vi "FPGA to RT to Host data stream trial.vi"() -> ()   [LabVIEW 2018]
uses:
  <vilib>/rvi/interface/nirviOpenFPGA/nirviOpenFPGA.xnode
  <vilib>/rvi/interface/nirviCloseFPGA/nirviCloseFPGA.xnode
  <vilib>/rvi/interface/nirviMethod/nirviMethod.xnode
  <vilib>/rvi/errors/niLvFpgaMergeErrorWithErrorCode.vi
  <vilib>/rvi/interface/nirviReadWriteControl/nirviReadWriteControl.xnode
  <vilib>/Utility/error.llb/Error Cluster From Error Code.vi
  <vilib>/rvi/interface/Simulation/niFpgaSimulationCallBeginRW.vi
  <vilib>/rvi/errors/niLvFpgaAdjustHostInterfaceError.vi
  <resource>/objmgr/ni.dex.rc
  <vilib>/dex/Flush And Wait Empty Condition.ctl
  <vilib>/FPGAPlugInAG/Dynamic/niLvFpga_Reset_Dynamic.vi
  <vilib>/FPGAPlugInAG/Dynamic/niLvFpga_Run_Dynamic.vi
  Type Defs/channelScalingTypes.ctl
  Type Defs/scalingMethods.ctl
  Type Defs/channelCalibration.ctl
  Type Defs/Data processing loop data.ctl
  Type Defs/FPGA reference.ctl
  FPGA Bitfiles/CompressorRigV2_CompressorFPGA_FPGAMain_VETZPGqYdEE.lvbitx
  FPGA/FPGA Main.vi
  <vilib>/FPGAPlugInAG/cRIO-9056/niLvFpga_Open_cRIO-9056.vi
  <vilib>/rvi/interface/common/dynamic/niFpgaDynamicAddResources.vi
  NiFpgaLv.dll
  <vilib>/FPGAPlugInAG/Dynamic/niLvFpga_ConfigureFifo_Dynamic.vi
  <vilib>/FPGAPlugInAG/Dynamic/niLvFpga_StartFifo_Dynamic.vi
  <vilib>/FPGAPlugInAG/Dynamic/niLvFpga_StopFifo_Dynamic.vi
  <vilib>/FPGAPlugInAG/Dynamic/niLvFpga_Close_Dynamic.vi
panel:
  out "Network available":bool
  in  "samples":u16=2500
  out "Channel count":u16
  in  "packet size":u32=610000
  in  "STOP":bool
  out "NS Capacity":T1(slide) caption="Network Stream capacity" scale=0.0..1220000.0
  out "Network fills":i32
  out "queue fills":i32
  out "lost packets":i32
  out "FIFO":T1(slide) caption="FIFO capacity" scale=0.0..762880.0
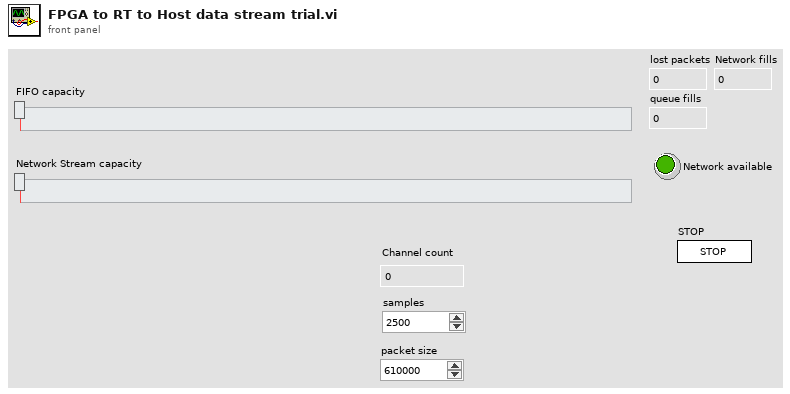
[diagram p1: front panel]
types:
  T1 = cluster{"Numeric":u32, "Numeric":u32, "Numeric":u32, "Numeric":u32}
  T2 = typedef "Data processing loop data.ctl" = cluster{"Parameters":cluster{"FPGA Ref":T3, "data stream":cluster{"data writer name":string, "NS write buffer size":i32, "NS Buffer length":u32}, "FIFO Depth":u32, "Channel controls":cluster{"FIFIO channel count":i32, "active indices":i16[], "active channels":i32, "channelScaling":T4[], "scanivalveCount":i32}, "safetyChannels":cluster{"oilP":u16, "airP":u16, "water":u16, "temperatures":cluster{"Oil pressure: 4":u16, "Enabled":bool, "warning temp":dbl, "limit temp":dbl, "Invert":bool}[]}}, "Variables":cluster{"Intermediary buffer":dbl[][], "buffer position":u32, "write loop counter":u16, "NS write trigger":u32, "NS Connection status":bool, "waiting for NS":bool, "labAmbient":cluster{"pressure":dbl, "temperature":dbl}, "scanivalvePorts":u16[], "scanivalvePressures":dbl[], "data stream":refnum<k21>}}
  T3 = typedef "FPGA reference.ctl" = refnum<k20>
  T4 = typedef "channelCalibration.ctl" = cluster{"index":u16, "active":bool, "channelType":T5, "module":u16, "terminal":u16, "channelName":string, "scalingMethod":T6, "scalingParameters":dbl[], "scaledUnits":string}
  T5 = typedef "channelScalingTypes.ctl" = enum16{"calculation", "measurement", "scanivalve", "output", "digital"}
  T6 = typedef "scalingMethods.ctl" = enum16{"none", "linear", "thermocouple", "polynomial", "encoder", "RTD"}
  T7 = cluster{"Value":u32, "read point":u32, "90":u32, "buffer depth":u32}
  T8 = typedef "Flush And Wait Empty Condition.ctl" = u8
  T9 = cluster{"Time":bool[], "Tcs":bool[], "RTDs":bool[], "HS VI":bool[], "AI":bool[], "LS VI":bool[], "Torque":bool[], "Pulser":bool[]}
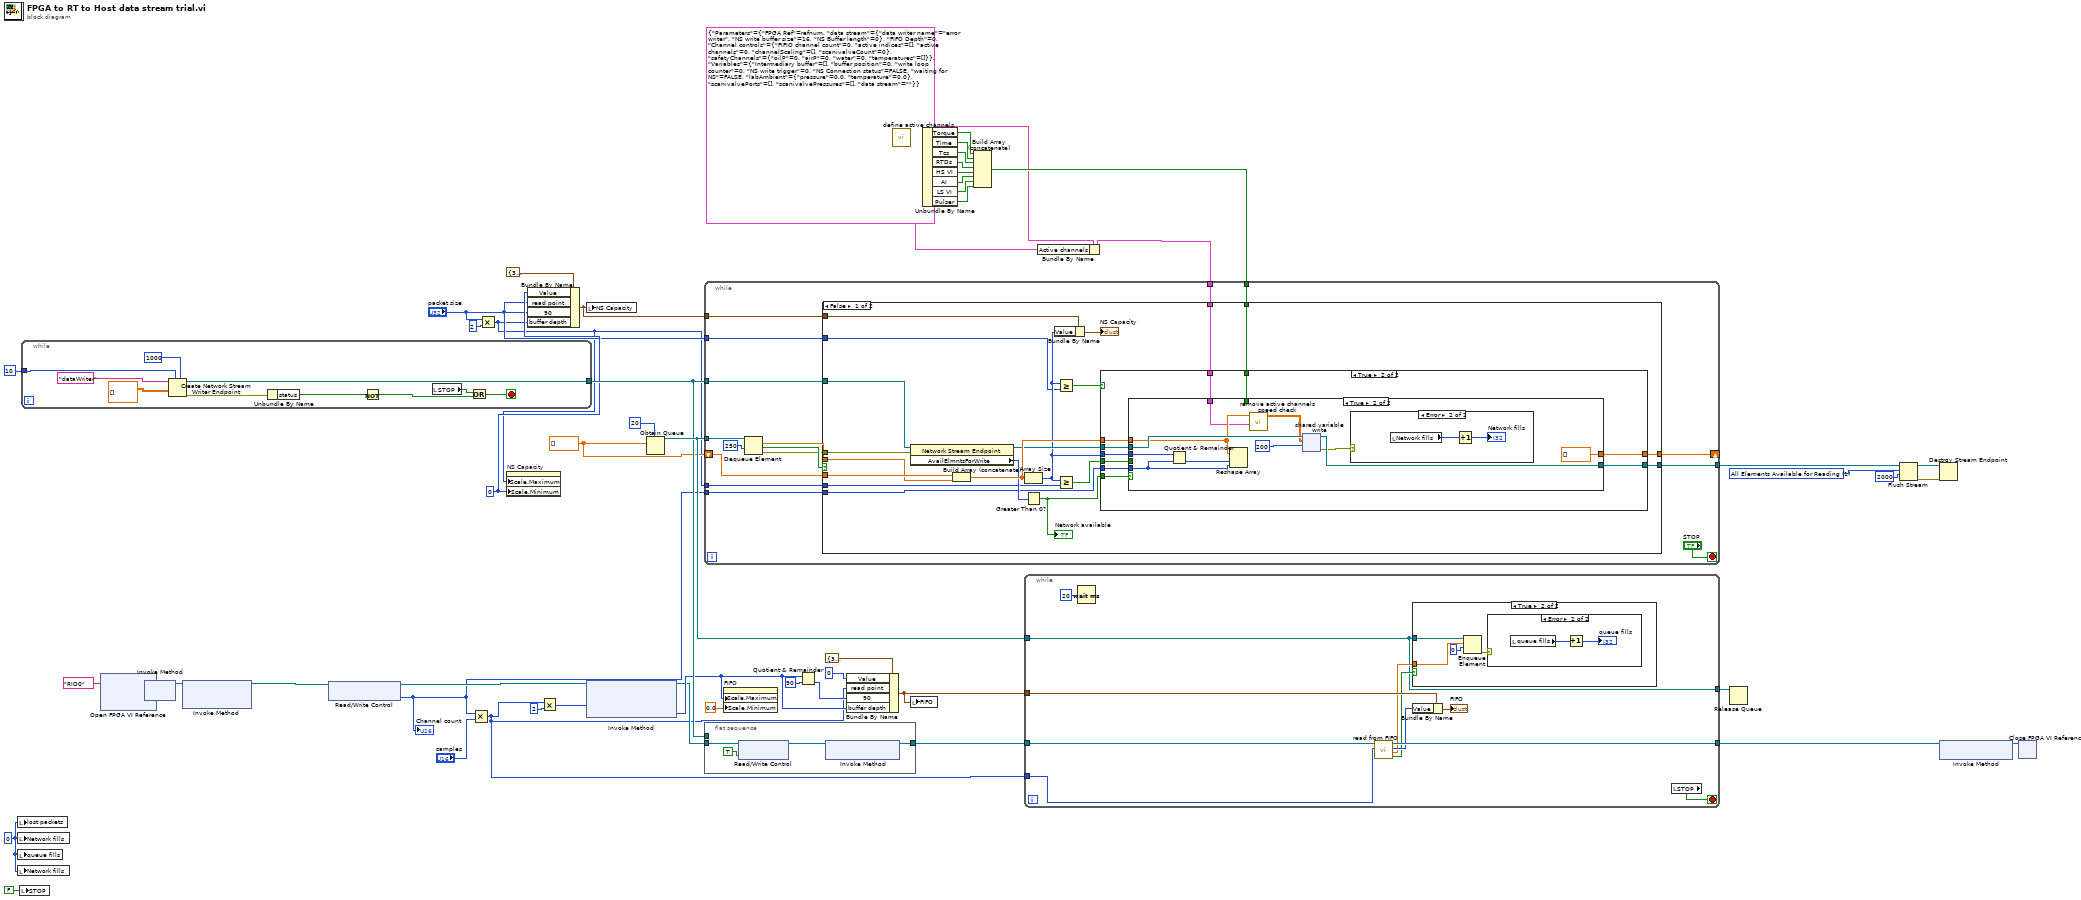
[diagram p0: block diagram]
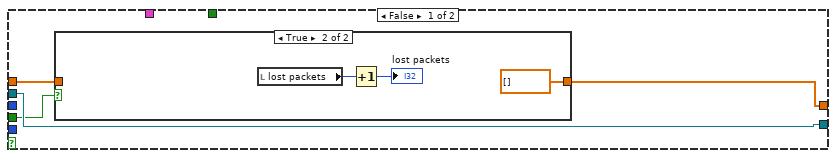
[diagram p3: hidden frame]
diagram:
  w24 = u32 0 ("Value")
  w23 = 0 ("Network fills")
  w28 = sgl[] [] ("Array")
  w41 = T8 1 items=["All Elements Read From Stream", "All Elements Available for Reading"] ("wait condition")
  n1 = local write "lost packets"(w23) -> ()
  n2 = local write "Network fills"(w23) -> ()
  n3 = local write "queue fills"(w23) -> ()
  n4 = local write "Network fills"(w23) -> ()
  n5 = local write "STOP"(FALSE ("STOP")) -> ()
  n6 = while {
    tunnel: [w59] -> w33
    tunnel: 10 ("writer buffer size") -> [w58]
    stop <- w57 stop-if-true
    n7 = Create Network Stream Writer Endpoint(5:1000 ("timeout in ms (-1)"), 7:w58, 9:sgl[][] [] ("Array"), 11:"dataWriter" ("writer name")) -> (0:w61:errorcluster, 3:w59:refnum<k21>)  [unwired: 3 in]
    n8 = Unbundle By Name(w61) -> ("status"=w55:bool)
    n9 = Not(x=w55) -> (.not. x?=w54:bool)
    n10 = local read "STOP"() -> (w56:bool)
    n11 = Or(x=w56, y=w54) -> (x .or. y?=w57:bool)
  }
  n12 = xnode "Open FPGA VI Reference"("resource name"=tag "RIO0") -> ("FPGA VI Reference Out"=w51:refnum<k20>)  [unwired: 1 in, 1 out]
  n13 = xnode "Invoke Method"("FPGA VI Reference In"=w51) -> ("FPGA VI Reference Out"=w22:refnum<k20>)  [unwired: 1 in, 1 out]
  n14 = xnode "Invoke Method"("FPGA VI Reference In"=w22) -> ("FPGA VI Reference Out"=w21:refnum<k20>)  [unwired: 2 in, 1 out]
  n15 = xnode "Read/Write Control"("FPGA VI Reference In"=w21) -> ("FPGA VI Reference Out"=w20:refnum<k20>, "Total channel count"=w14:i32)  [unwired: 1 in, 1 out]
  "Channel count" <- w14
  n16 = Multiply(x=w14, y="samples") -> (x*y=w17:i32)
  n17 = Multiply(x="packet size", y=u32 2) -> (x*y=w13:u32)
  n18 = property on="NS Capacity" class="Slide (strict)"("Scale.Maximum"=w13, "Scale.Minimum"=w24) -> ()  [unwired: 2 in, 2 out]
  n19 = Bundle By Name(cluster=T7 {"Value"=3, "read point"=8, "90"=8, "buffer depth"=10} ("Buffer"), "Value"=w24, "read point"="packet size", "90"="packet size", "buffer depth"=w13) -> (w31:T7)
  n20 = Multiply(x=w17, y=u32 2) -> (x*y=w26:u32)
  n21 = local write "NS Capacity"(w31) -> ()
  n22 = xnode "Invoke Method"("FPGA VI Reference In"=w20, "Requested Depth"=w26) -> ("FPGA VI Reference Out"=w19:refnum<k20>, "Actual Depth"=w29:u32)  [unwired: 1 in, 1 out]
  n23 = Obtain Queue(max queue size (-1, unlimited)=20, element data type=w28) -> (queue out=w35:refnum<queue>)  [unwired: 3 in, 2 out]
  n24 = flat-sequence {
    tunnel: [w66] -> w50
    tunnel: w33 -> [_]
    tunnel: w19 -> [w65]
    frame #0 {
      n25 = xnode "Read/Write Control"("FPGA VI Reference In"=w65, "Stop acquire"=TRUE) -> ("FPGA VI Reference Out"=w64:refnum<k20>)  [unwired: 1 in, 1 out]
      n26 = xnode "Invoke Method"("FPGA VI Reference In"=w64) -> ("FPGA VI Reference Out"=w66:refnum<k20>)  [unwired: 1 in, 1 out]
    }
  }
  n27 = property on="FIFO" class="Slide (strict)"("Scale.Maximum"=w29, "Scale.Minimum"=0.0 ("Scale.Range:Minimum")) -> ()  [unwired: 2 in, 2 out]
  n28 = Quotient & Remainder(x=w29, y=u32 90) -> (floor(x/y)=w44:u32)  [unwired: 1 out]
  n29 = Bundle By Name(cluster=T7 {"Value"=3, "read point"=8, "90"=8, "buffer depth"=10} ("Buffer"), "Value"=u32 0, "read point"=w17, "90"=w44, "buffer depth"=w29) -> (w43:T7)
  n30 = call "define active channels.vi"() -> ("Active channels"=w1:T9)  [unwired: 9 in, 2 out]
  n31 = local write "FIFO"(w43) -> ()
  n32 = Unbundle By Name(w1) -> ("Torque"=w12:bool[], "Time"=w11:bool[], "Tcs"=w10:bool[], "RTDs"=w9:bool[], "HS VI"=w8:bool[], "AI"=w7:bool[], "LS VI"=w6:bool[], "Pulser"=w5:bool[])
  n33 = Build Array (concatenate)(w12, w11, w10, w9, w8, w7, w6, w5) -> (w4:bool[])
  n34 = while {
    tunnel: w50 -> [w67]
    tunnel: [w77] -> w52
    tunnel: w17 -> [w76]
    tunnel: w43 -> [w75]
    tunnel: w35 -> [w70]
    tunnel: [w70] -> w34
    stop <- w69 stop-if-true
    n35 = Wait (ms)(milliseconds to wait=u32 20) -> ()  [unwired: 1 out]
    n36 = call "read from FIFO.vi"("Read size"=w76, "Refnum in"=w67) -> ("data read?"=w72:bool, "Data"=w71:sgl[], "FIFO level"=w73:u32, "FPGA VI Reference Out"=w77:refnum<k20>)  [unwired: 6 in]
    n37 = case shown="True" w72 {
      tunnel: w70 -> [_ w81]
      tunnel: w71 -> [_ w80]
      frame False {
      }
      frame True {
        n38 = Enqueue Element(queue=w81, element=w80, timeout in ms (-1)=0) -> (error out=w78:errorcluster)  [unwired: 1 in, 2 out]
        n39 = case shown="Error" w78 {
          frame No Error {
          }
          frame Error {
            n40 = local read "queue fills"() -> (w83:i32)
            n41 = Increment(x=w83) -> (x+1=→"queue fills":i32)
          }
        }
      }
    }
    n42 = Bundle By Name(cluster=w75, "Value"=w73) -> (→"FIFO":T7)
    n43 = local read "STOP"() -> (w69:bool)
  }
  n44 = Bundle By Name(cluster=T2 {"Parameters"={"FPGA Ref"=refnum, "data stream"={"data writer name"="error writer", "NS write buffer size"=16, "NS Buffer length"=0}, "FIFO Depth"=0, "Channel controls"={"FIFIO channel count"=0, "active indices"=[], "active channels"=0, "channelScaling"=[], "scanivalveCount"=0}, "safetyChannels"={"oilP"=0, "airP"=0, "water"=0, "temperatures"=[]}}, "Variables"={"Intermediary buffer"=[], "buffer position"=0, "write loop counter"=0, "NS write trigger"=0, "NS Connection status"=FALSE, "waiting for NS"=FALSE, "labAmbient"={"pressure"=0.0, "temperature"=0.0}, "scanivalvePorts"=[], "scanivalvePressures"=[], "data stream"=""}} ("Data"), "Active channels"=w1) -> (w2:T2)
  n45 = while {
    tunnel: w33 -> [w91]
    tunnel: [w99] -> w37
    tunnel: w35 -> [w98]
    tunnel: w31 -> [w89]
    shift-right: [w92] -> _
    shift-left: w28 -> [w94]
    tunnel: "packet size" -> [w88]
    tunnel: w13 -> [w87]
    tunnel: w14 -> [w86]
    tunnel: w4 -> [w85]
    tunnel: w2 -> [w84]
    stop <- "STOP" stop-if-true
    n46 = Dequeue Element(queue=w98, timeout in ms (-1)=250) -> (element=w93:sgl[], timed out?=w96:bool, error out=w90:errorcluster)  [unwired: 1 in, 1 out]
    n47 = case shown="False" w96 {
      tunnel: [w119 w153] -> w99
      tunnel: w94 -> [w118 w154]
      tunnel: w93 -> [w102 _]
      tunnel: [w111 w154] -> w92
      tunnel: w91 -> [w116 w153]
      tunnel: w90 -> [w115 _]
      tunnel: w89 -> [w109 _]
      tunnel: w88 -> [w105 _]
      tunnel: w87 -> [w104 _]
      tunnel: w86 -> [w103 _]
      tunnel: w85 -> [w101 _]
      tunnel: w84 -> [w100 _]
      frame False {
        n48 = property class="Network Stream Endpoint"(reference=w116, error in=w115) -> (reference out=w114:refnum<k21>, "AvailElmntsForWrite"=w107:i32)  [unwired: 1 out]
        n49 = Build Array (concatenate)(w118, w102) -> (w117:sgl[])
        n50 = Array Size(array=w117) -> (size(s)=w106:i32)
        n51 = Greater Than 0?(x=w107) -> (x > 0?=w112:bool)
        "Network available" <- w112
        n52 = Bundle By Name(cluster=w109, "Value"=w106) -> (→"NS Capacity":T7)
        n53 = Greater Or Equal?(x=w106, y=w105) -> (x >= y?=w113:bool)
        n54 = Greater Or Equal?(x=w106, y=w104) -> (x >= y?=w108:bool)
        n55 = case shown="True" w113 {
          tunnel: [w121 w131] -> w119
          tunnel: w117 -> [w120 w130]
          tunnel: w114 -> [w121 w129]
          tunnel: w112 -> [_ w128]
          tunnel: [w120 w127] -> w111
          tunnel: w108 -> [_ w126]
          tunnel: w106 -> [_ w125]
          tunnel: w103 -> [_ w124]
          tunnel: w101 -> [_ w123]
          tunnel: w100 -> [_ w122]
          frame False {
          }
          frame True {
            n56 = case shown="True" w128 {
              tunnel: w130 -> [w132 w142]
              tunnel: w129 -> [w135 w150]
              tunnel: [w135 w148] -> w131
              tunnel: [w133 sgl[] []] -> w127
              tunnel: w126 -> [w134 _]
              tunnel: w125 -> [_ w144]
              tunnel: w124 -> [_ w143]
              tunnel: w123 -> [_ _]
              tunnel: w122 -> [_ w140]
              frame False {
                n57 = case shown="True" w134 {
                  tunnel: [w136 sgl[] []] -> w133
                  tunnel: w132 -> [w136 _]
                  frame False {
                  }
                  frame True {
                    n58 = local read "lost packets"() -> (w139:i32)
                    n59 = Increment(x=w139) -> (x+1=→"lost packets":i32)
                  }
                }
              }
              frame True {
                n60 = Quotient & Remainder(x=w144, y=w143) -> (floor(x/y)=w145:i32)  [unwired: 1 out]
                n61 = Reshape Array(w142, w145, w143) -> ()  [unwired: 1 out]
                n62 = call "remove active channels speed check.vi"("Data"=w140, "raw data"=w142) -> ("Active channels"=w141:sgl[][])  [unwired: 8 in, 1 out]
                n63 = shared-variable-write(w150, w141, 200 ("timeout ms (-1)")) -> (w148:refnum<k21>, w147:errorcluster)  [unwired: 1 in, 1 out]
                n64 = case shown="Error" w147 {
                  frame No Error {
                  }
                  frame Error {
                    n65 = local read "Network fills"() -> (w152:i32)
                    n66 = Increment(x=w152) -> (x+1=→"Network fills":i32)
                  }
                }
              }
            }
          }
        }
      }
      frame True {
      }
    }
  }
  n67 = Release Queue(queue=w34) -> ()  [unwired: 2 in, 3 out]
  n68 = Flush Stream(9:2000 ("timeout in ms (-1)"), 10:w41, 11:w37) -> (0:w38:errorcluster, 3:w40:refnum<k21>)  [unwired: 1 in, 1 out]
  n69 = Destroy Stream Endpoint(8:w38, 11:w40) -> ()  [unwired: 1 out]
  n70 = xnode "Invoke Method"("FPGA VI Reference In"=w52) -> ("FPGA VI Reference Out"=w49:refnum<k20>)  [unwired: 1 in, 1 out]
  n71 = xnode "Close FPGA VI Reference"("FPGA VI Reference In"=w49) -> ()  [unwired: 1 in, 1 out]
